vi "cRIO.vi"() -> ()   [LabVIEW 2015]
uses:
  <vilib>/FPGAPlugInAG/cRIO-9113/niLvFpga_Open_cRIO-9113.vi
  <vilib>/rvi/interface/common/dynamic/niFpgaDynamicAddResources.vi
  <vilib>/Utility/error.llb/Error Cluster From Error Code.vi
  <vilib>/FPGAPlugInAG/Dynamic/niLvFpga_Run_Dynamic.vi
  <vilib>/rvi/interface/common/niFpgaWaitOnOcc.vi
  <vilib>/rvi/errors/niLvFpgaAdjustHostInterfaceError.vi
  <vilib>/FPGAPlugInAG/Dynamic/niLvFpga_Close_Dynamic.vi
  <vilib>/rvi/interface/nirviOpenFPGA/nirviOpenFPGA.xnode
  FPGA Bitfiles/DW40ticks_FPGATarget_Fpga_vnTk4tnBuVA.lvbitx
  Fpga.vi
  <vilib>/rvi/interface/nirviMethod/nirviMethod.xnode
  <vilib>/rvi/interface/nirviReadWriteControl/nirviReadWriteControl.xnode
  <vilib>/rvi/interface/nirviCloseFPGA/nirviCloseFPGA.xnode
  <vilib>/FPGAPlugInAG/Dynamic/niLvFpga_StartFifo_Dynamic.vi
  <vilib>/rvi/errors/niLvFpgaMergeErrorWithErrorCode.vi
  <vilib>/FPGAPlugInAG/Dynamic/niLvFpga_ConfigureFifo_Dynamic.vi
  <vilib>/FPGAPlugInAG/Dynamic/niLvFpga_ReadFifo_Dynamic.vi
  NiFpgaLv.dll
  <vilib>/rvi/interface/Simulation/niFpgaSimulationCallBeginRW.vi
panel:
  out "error out":errorcluster
  out "s? t:f":u8
  out "Timed Out?":bool
  in  "stop":bool
  out "Elements Remaining":u32
  out "Actual Depth":u32
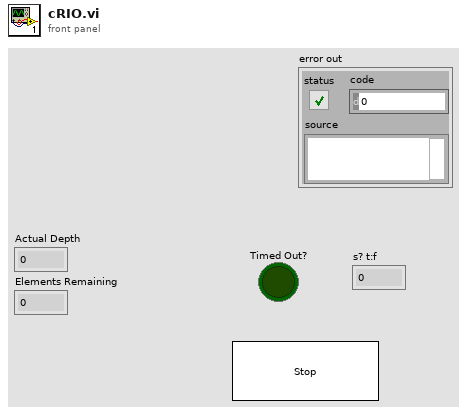
[diagram p1: front panel]
types:
  T1 = enum16{"open", "open or create", "create or replace", "create", "open (read-only)"}
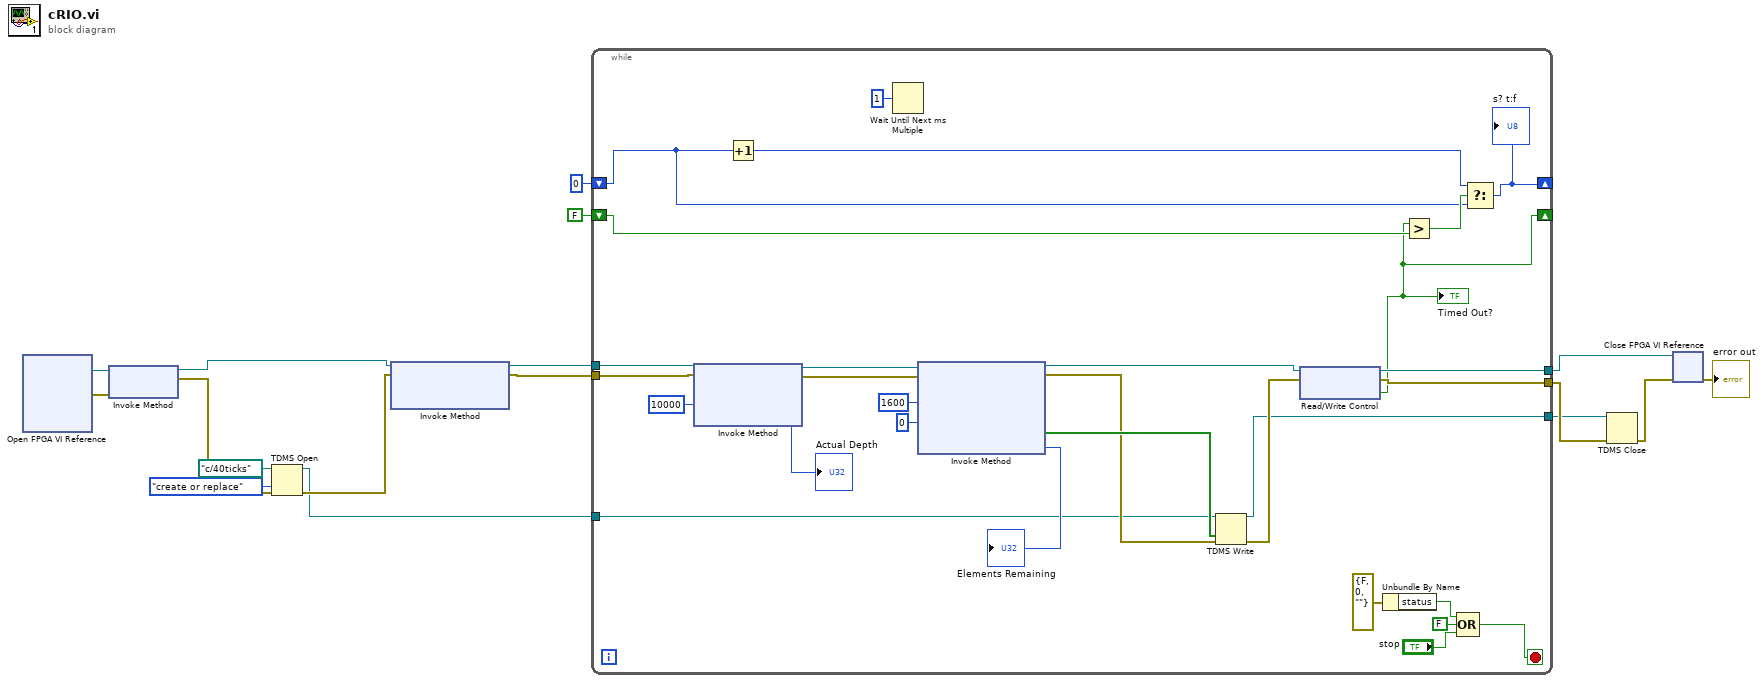
[diagram p0: block diagram]
diagram:
  n1 = xnode "Open FPGA VI Reference"() -> ("FPGA VI Reference Out"=w17:refnum<k20>, "error out"=w16:errorcluster)  [unwired: 2 in]
  n2 = xnode "Invoke Method"("FPGA VI Reference In"=w17, "error in"=w16) -> ("FPGA VI Reference Out"=w14:refnum<k20>, "error out"=w15:errorcluster)
  n3 = TDMS Open(8:w15, 10:T1."create or replace" ("operation (0:open)"), 11:path "c:/40ticks" ("file path")) -> (0:w13:errorcluster, 3:w8:refnum<k34>)  [unwired: 4 in]
  n4 = xnode "Invoke Method"("FPGA VI Reference In"=w14, "error in"=w13) -> ("FPGA VI Reference Out"=w12:refnum<k20>, "error out"=w11:errorcluster)  [unwired: 1 in]
  n5 = while {
    tunnel: w12 -> [w46]
    tunnel: w11 -> [w45]
    tunnel: w8 -> [w35]
    tunnel: [w31] -> w7
    tunnel: [w27] -> w6
    tunnel: [w30] -> w4
    shift-right: [w25] -> _
    shift-left: FALSE ("Timed Out?") -> [w26]
    shift-right: [w21] -> _
    shift-left: u8 0 -> [w23]
    stop <- w29 stop-if-true
    n6 = xnode "Invoke Method"("FPGA VI Reference In"=w46, "error in"=w45, "Requested Depth"=u32 10000) -> ("FPGA VI Reference Out"=w42:refnum<k20>, "error out"=w41:errorcluster, "Actual Depth"=→"Actual Depth":u32)
    n7 = Increment(x=w23) -> (x+1=w22:u8)
    n8 = Wait Until Next ms Multiple(millisecond multiple=u32 1) -> ()  [unwired: 1 out]
    n9 = xnode "Invoke Method"("FPGA VI Reference In"=w42, "error in"=w41, "Number of Elements"=u32 1600, "Timeout (ms)"=0) -> ("FPGA VI Reference Out"=w33:refnum<k20>, "error out"=w36:errorcluster, "Data"=w37:bool[], "Elements Remaining"=→"Elements Remaining":u32)
    n10 = TDMS Write(0:w35, 9:w37, 11:w36) -> (4:w30:refnum<k34>, 15:w34:errorcluster)  [unwired: 3 in, 2 out]
    n11 = xnode "Read/Write Control"("FPGA VI Reference In"=w33, "error in"=w34) -> ("FPGA VI Reference Out"=w31:refnum<k20>, "error out"=w27:errorcluster, "Timed Out?"=w25:bool)
    "Timed Out?" <- w25
    n12 = Unbundle By Name(errorcluster {"status"=FALSE, "code"=0, "source"=""} ("input cluster")) -> ("status"=w20:bool)
    n13 = Greater?(x=w25, y=w26) -> (0:w24:bool)
    n14 = Compound Arithmetic op=OR(w20, FALSE ("value"), "stop") -> (w29:bool)
    n15 = Select(t=w22, s=w24, f=w23) -> (s? t:f=w21:u8)
    "s? t:f" <- w21
  }
  n16 = TDMS Close(8:w6, 11:w4) -> (0:w5:errorcluster)  [unwired: 1 out]
  n17 = xnode "Close FPGA VI Reference"("FPGA VI Reference In"=w7, "error in"=w5) -> ("error out"=→"error out":errorcluster)
